vi "GOMDBTS2048 weighting Get Factors.vi"(8 "error in (no error)":errorcluster, 10 "parameter":i32, 11 "handle":i32) -> (0 "error out":errorcluster, 2 "function return":i32, 3 "weighting value":dbl, 4 "to WL":dbl, 5 "from WL":dbl)   [LabVIEW 2015, in "GOMDBTS2048.lvlib"]
doc: "GOBTS2048DLL int __stdcall GOMDBTS2048_integralGetWeightingFactors(int handle, int parameter, double* value);"
uses:
  GOMDBTS2048.lvlib
  runtime/GOMDBTS2048.dll
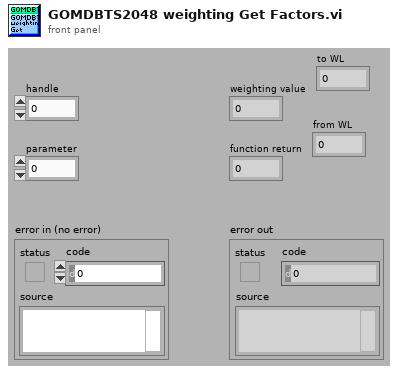
[diagram p1: front panel]
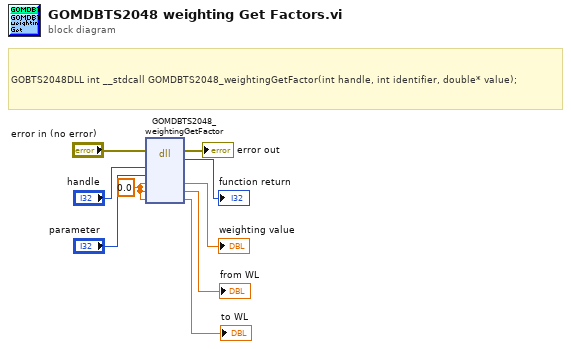
[diagram p0: block diagram]
diagram:
  w3 = 0.0 ("weighting value")
  # "GOBTS2048DLL int __stdcall GOMDBTS2048_weightingGetFactor(int handle, int identifier, double* value);"
  n1 = dll-call lib="C:/Users/rkoch/Documents/GO_Library/runtime/GOMDBTS2048.*" fn="GOMDBTS2048_weightingGetFactor"(error in="error in (no error)", "handle"="handle", "parameter"="parameter", "weighting value"=w3, "fromWL"=w3, "toWl"=w3) -> (error out=→"error out":errorcluster, "return type"=→"function return":i32, "weighting value"=→"weighting value":dbl, "fromWL"=→"from WL":dbl, "toWl"=→"to WL":dbl)  [unwired: 4 in, 1 out]
